vi "Read BFECC Automation Path.vi"(8 "error in (no error)":errorcluster, 11 "BFECC in":refnum<class "BFECC.lvclass">) -> (0 "error out":errorcluster, 2 "BFECC Automation Path":path, 3 "BFECC out":refnum<class "BFECC.lvclass">)   [LabVIEW 2018, in "BFECC.lvlib" / "BFECC.lvclass"]
uses:
  BFECC.lvclass
  BFECC.lvclass/BFECC.ctl
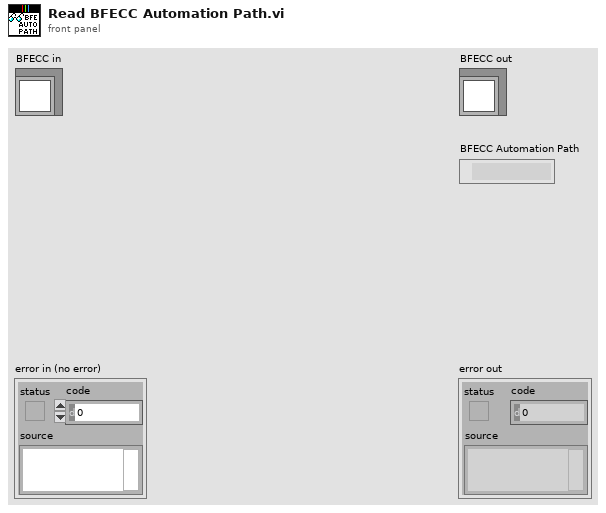
[diagram p1: front panel]
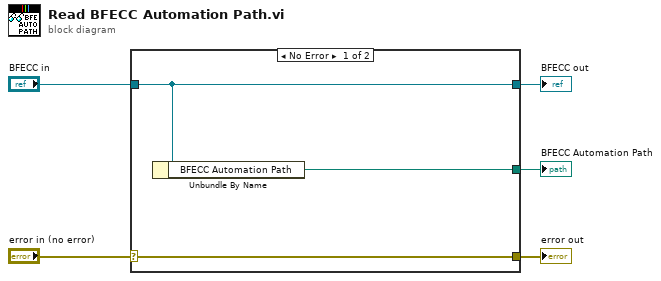
[diagram p0: block diagram]
diagram:
  n1 = case shown="No Error" "error in (no error)" {
    selector: "error in (no error)" -> [w8 w9]
    tunnel: [w8 w9] -> w4
    tunnel: [w7 w10] -> w2
    tunnel: "BFECC in" -> [w7 w10]
    tunnel: [w6 _] -> w1
    frame No Error {
      n2 = Unbundle By Name(w7) -> ("BFECC Automation Path"=w6:path)
    }
    frame Error {
    }
  }
  "error out" <- w4
  "BFECC out" <- w2
  "BFECC Automation Path" <- w1
